vi "Get all Channel Settings File Names.vi"() -> (3 "Channel Settings Files":string[](array[string]))   [LabVIEW 2019, in "Settings Editor.lvlib"]
uses:
  Settings Editor.lvlib
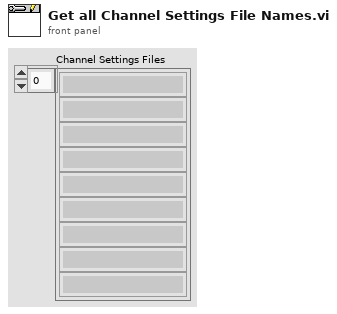
[diagram p1: front panel]
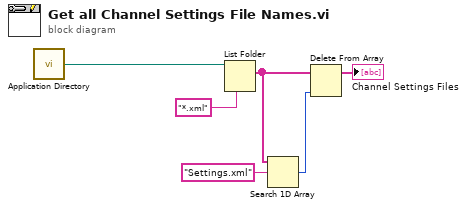
[diagram p0: block diagram]
diagram:
  n1 = call <vilib>:"Application Directory.vi"() -> ("Application Directory"=w5:path)
  n2 = List Folder(path=w5, pattern="*.xml") -> (filenames=w3:string[])  [unwired: 2 in, 3 out]
  n3 = Search 1D Array(1D array=w3, element="Settings.xml") -> (index of element=w2:i32)  [unwired: 1 in]
  n4 = Delete From Array(array=w3, index=w2) -> (array with subset deleted=→"Channel Settings Files":string[])  [unwired: 1 in, 1 out]
